vi "Add Boost Stage.vi"(8 "error in (no error)":errorcluster, 10 "Stage Name":string, 11 "Shot Section Item Ref":T1=18446744073709551615 format="%.0x") -> (0 "error out":errorcluster, 3 "Shot Section Item Ref dup":T1=18446744073709551615 format="%.0x")   [LabVIEW 2015, in "Fuel Injection Addon System Explorer.lvlib"]
uses:
  Fuel Injection Addon System Explorer.lvlib
  <vilib>/NI Veristand/Custom Device API/Custom Device Item Ref.ctl
  Shared/Types/Analysis.Channels.Select.ctl
  Shared/Constants.vi
  Shared/Fuel Injection Addon Shared.lvlib
  <vilib>/NI VeriStand/Custom Device API/Custom Device API.lvlib
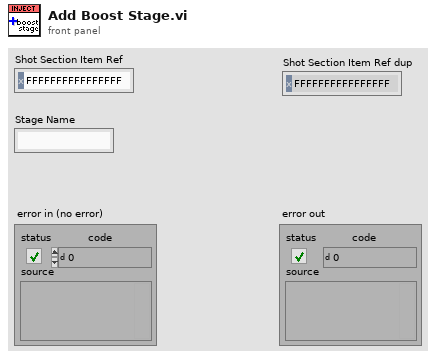
[diagram p1: front panel]
types:
  T1 = typedef "Custom Device API.lvlib/Custom Device Item Ref.ctl" = u64
  T2 = typedef "Fuel Injection Addon Shared.lvlib/Analysis.Channels.Select.ctl" = cluster{"Pull In Time":bool, "Pull In Max Current":bool, "Hold In Time":bool, "Hold In Max Current":bool, "Hold In Min Current":bool, "Hold In Avg Current":bool, "Hold In Avg Max Current":bool, "Hold In Avg Min Current":bool, "Hold In Max Volt":bool, "Hold In Min Volt":bool, "Hold In Avg Volt":bool, "Hold In Avg Max Volt":bool, "Hold In Avg Min Volt":bool, "Off Time":bool, "Off-Stage Max Current":bool, "Off-Stage Min Current":bool, "Off-Stage Avg Current":bool, "Total Voltage Pulses":bool}
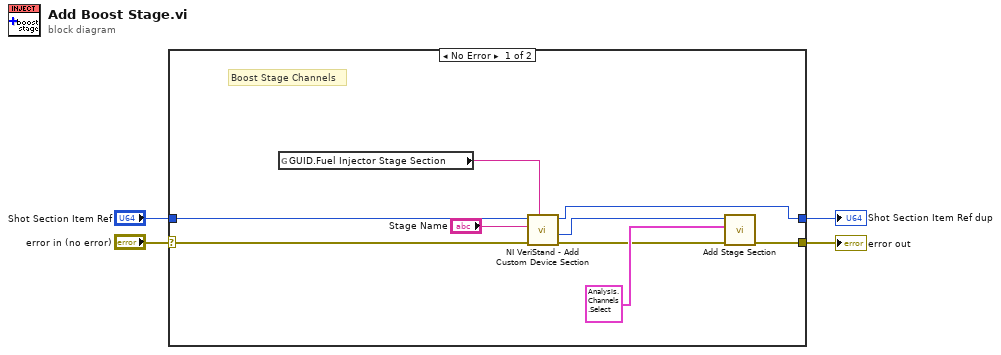
[diagram p0: block diagram]
diagram:
  n1 = case shown="No Error" "error in (no error)" {
    selector: "error in (no error)" -> [w11 w14]
    tunnel: "Shot Section Item Ref" -> [w10 w15]
    tunnel: [w5 w15] -> w2
    tunnel: [w13 w14] -> w1
    frame No Error {
      # "Boost Stage Channels"
      n2 = global read "Constants.vi" "GUID.Fuel Injector Stage Section"() -> (w12:string)
      n3 = call <vilib>:"NI VeriStand - Add Custom Device Section.vi"("GUID (Default Section)"=w12, "error in (no error)"=w11, "Section Name"="Stage Name", "Parent Ref in"=w10) -> ("error out"=w7:errorcluster, "Section Ptr"=w6:T1, "Parent Ref out"=w5:T1)  [unwired: 4 in, 1 out]
      n4 = call "Add Stage Section.vi"("error in (no error)"=w7, "Analysis Options"=T2 {"Pull In Time"=TRUE, "Pull In Max Current"=TRUE, "Hold In Time"=TRUE, "Hold In Max Current"=TRUE, "Hold In Min Current"=TRUE, "Hold In Avg Current"=TRUE, "Hold In Avg Max Current"=TRUE, "Hold In Avg Min Current"=TRUE, "Hold In Max Volt"=TRUE, "Hold In Min Volt"=TRUE, "Hold In Avg Volt"=TRUE, "Hold In Avg Max Volt"=TRUE, "Hold In Avg Min Volt"=TRUE, "Off Time"=TRUE, "Off-Stage Max Current"=TRUE, "Off-Stage Min Current"=TRUE, "Off-Stage Avg Current"=TRUE, "Total Voltage Pulses"=TRUE}, "Shot Section reference in"=w6) -> ("error out"=w13:errorcluster)  [unwired: 7 in, 1 out]
    }
    frame Error {
    }
  }
  "error out" <- w1
  "Shot Section Item Ref dup" <- w2
